vi "util.get.between.string.vi"(10 "search string/char (-)":string, 11 "String in":string) -> (3 "String out":string)   [LabVIEW 2021]
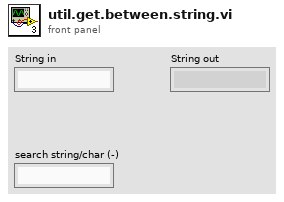
[diagram p1: front panel]
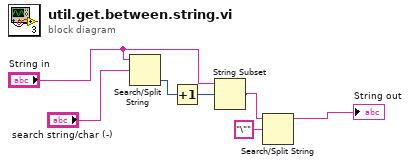
[diagram p0: block diagram]
diagram:
  n1 = Search/Split String(string="String in", search string/char (-)="search string/char (-)") -> (offset of match=w2:i32)  [unwired: 1 in, 2 out]
  n2 = Increment(x=w2) -> (x+1=w3:i32)
  n3 = String Subset(string="String in", offset (0)=w3) -> (substring=w5:string)  [unwired: 1 in]
  n4 = Search/Split String(string=w5, search string/char (-)="\"") -> (substring before match=→"String out":string)  [unwired: 1 in, 2 out]
